vi "Check outlier for merge.vi"(10 "Line 2":cluster{"Points":cluster{"X":dbl, "Y":dbl}[]}, 11 "Line 1":cluster{"Points":cluster{"X":dbl, "Y":dbl}[]}) -> (3 "Largest Outlier Distance":dbl)   [LabVIEW 2017]
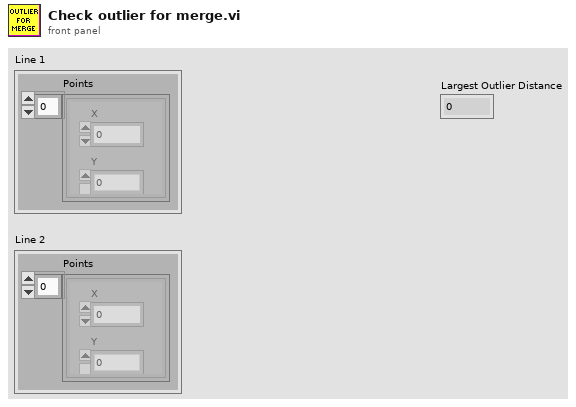
[diagram p1: front panel]
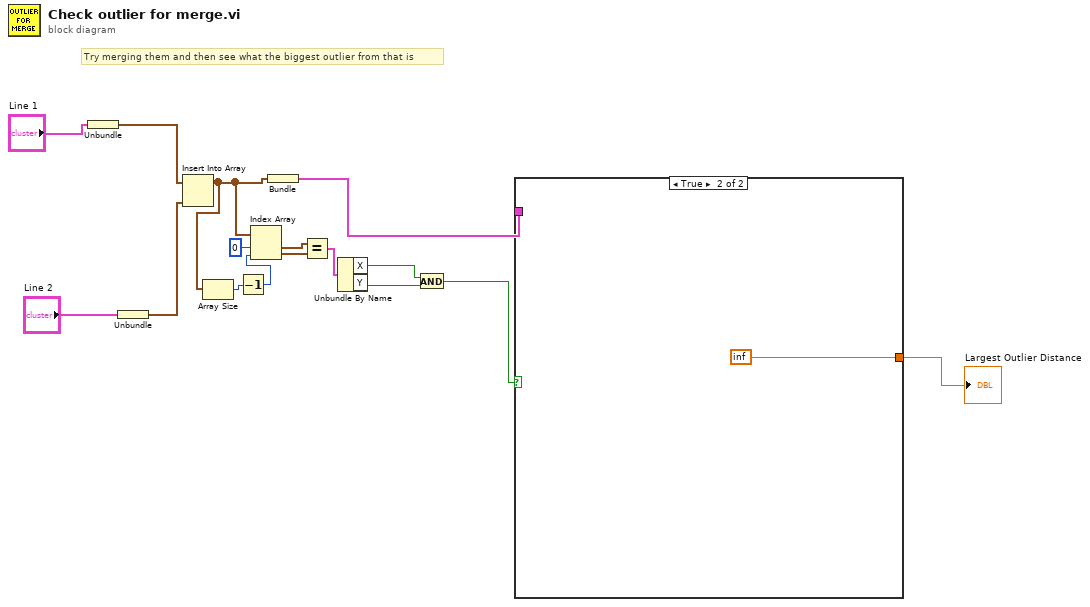
[diagram p0: block diagram]
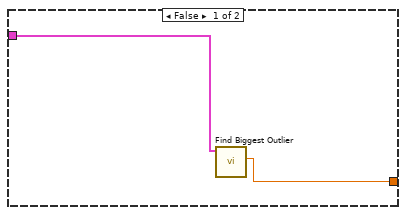
[diagram p2: hidden frame]
diagram:
  # "Try merging them and then see what the biggest outlier from that is"
  n1 = Unbundle("Line 1") -> ("Points"=w14:cluster{"X":dbl, "Y":dbl}[])
  n2 = Unbundle("Line 2") -> ("Points"=w13:cluster{"X":dbl, "Y":dbl}[])
  n3 = Insert Into Array(array=w14, new element=w13) -> (w11:cluster{"X":dbl, "Y":dbl}[])  [unwired: 1 in]
  n4 = Array Size(array=w11) -> (size(s)=w9:i32)
  n5 = Decrement(x=w9) -> (x-1=w10:i32)
  n6 = Index Array(array=w11, index #1=0 ("index"), index #2=w10) -> (element #1=w8:cluster{"X":dbl, "Y":dbl}, element #2=w7:cluster{"X":dbl, "Y":dbl})
  n7 = Bundle("Points"=w11) -> (w6:cluster{"Points":cluster{"X":dbl, "Y":dbl}[]})  [unwired: 1 in]
  n8 = Equal?(x=w8, y=w7) -> (x = y?=w4:cluster{"X":bool, "Y":bool})
  n9 = Unbundle By Name(w4) -> ("X"=w3:bool, "Y"=w2:bool)
  n10 = And(x=w3, y=w2) -> (x .and. y?=w1:bool)
  n11 = case shown="True" w1 {
    tunnel: w6 -> [w17 _]
    tunnel: [w18 inf] -> w5
    frame False {
      n12 = call "Find Biggest Outlier.vi"("Line with outlier"=w17) -> ("Outlier Amount"=w18:dbl)  [unwired: 9 in, 1 out]
    }
    frame True {
    }
  }
  "Largest Outlier Distance" <- w5
